vi "多参数测量数据读取.vi"(8 "Error in":errorcluster caption="Error in (no error)", 11 "探头选择":u16(ring)=9 items=["氨氮"=3, "水温"=9, "pH值"=10, "溶解氧"=11, "电导率"=12, "浊度"=13, "叶绿素a"=14, "藻密度"=15, "蓝绿藻"=16, "氧化还原电位"=17, "溶解氧%"=18, "盐度"=19]) -> (0 "error out":errorcluster, 2 "添加的数组":string[][](array[string]), 3 "测量数据块":T1)   [LabVIEW 2016, in "斯坦道原位多参数.lvlib"]
panel:
  in  "测量数据区":i32(listbox)
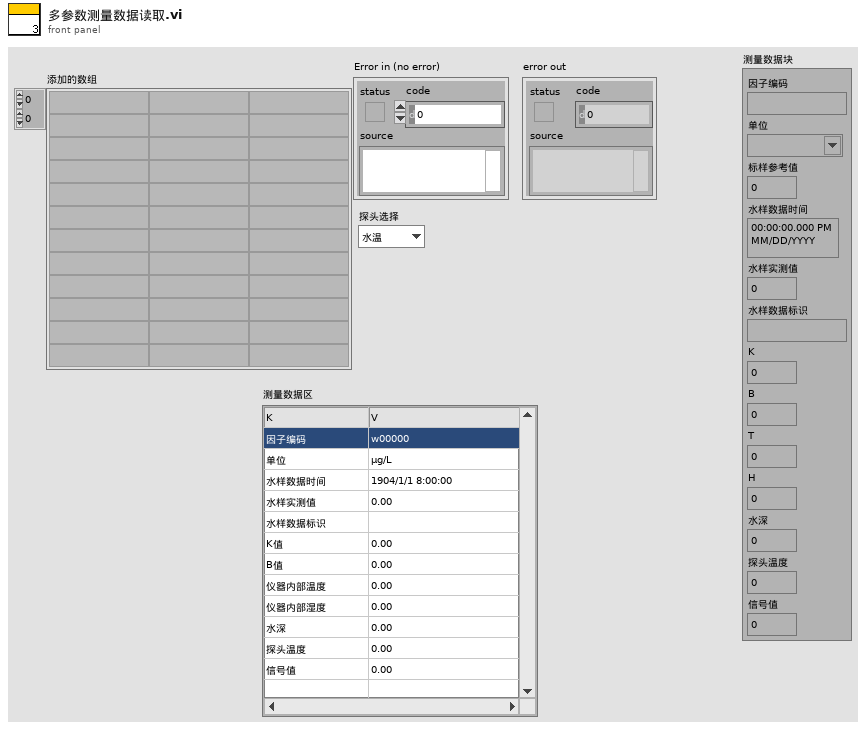
[diagram p1: front panel]
types:
  T1 = cluster{"因子编码":string, "单位":string, "标样参考值":sgl, "水样数据时间":timestamp, "水样实测值":sgl, "水样数据标识":string, "K":sgl, "B":sgl, "T":sgl, "H":sgl, "水深":sgl, "探头温度":sgl, "信号值":sgl}
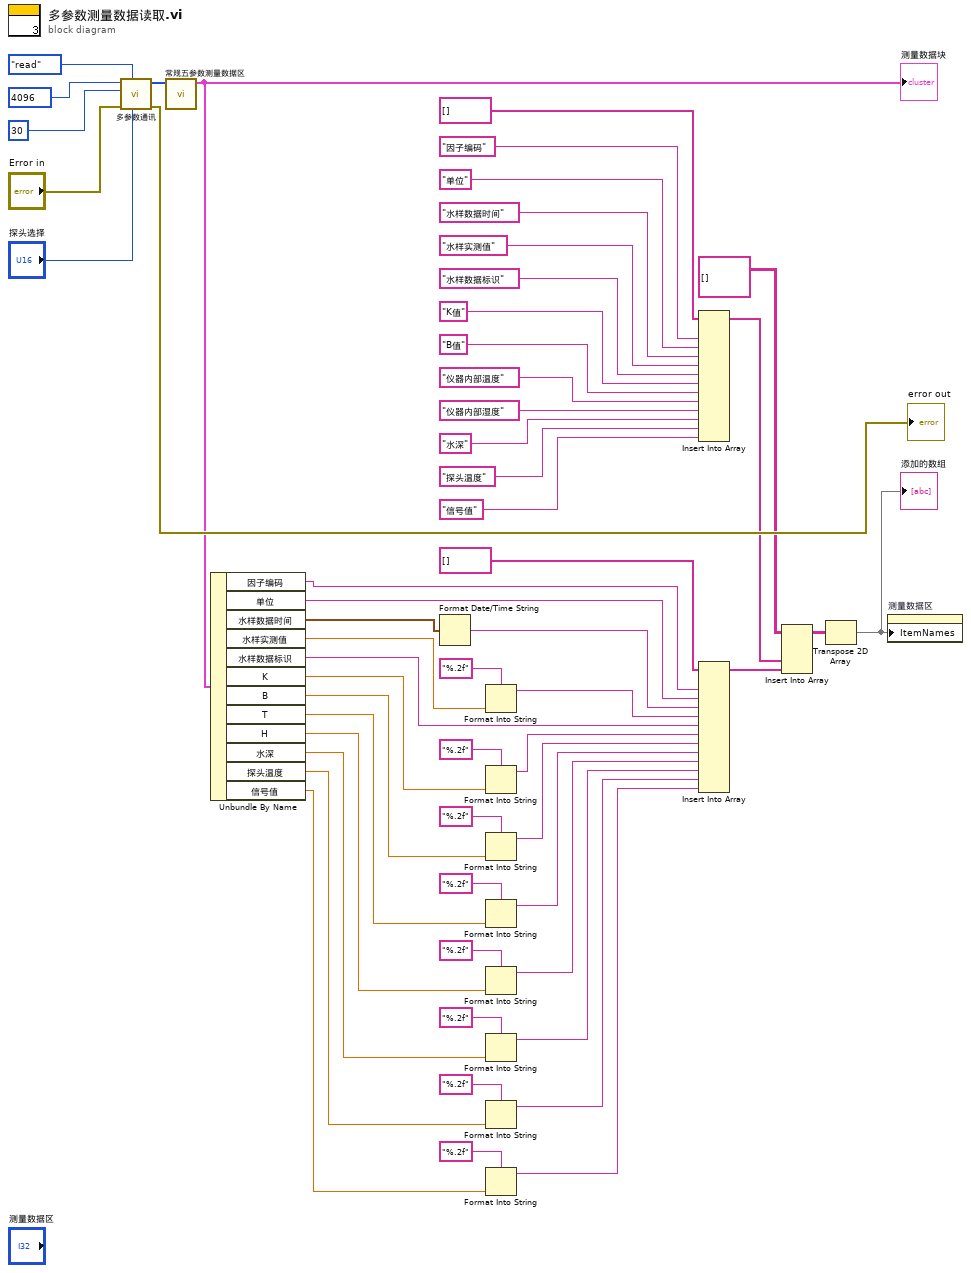
[diagram p0: block diagram]
diagram:
  n1 = call "多参数通讯.vi"("Slave ID"="探头选择", "STEP"=enum16{"open", "read", "write", "close"}."read", "Error in"="Error in", "quantity"=u16 30, "starting address"=u16 4096) -> ("error out"=→"error out":errorcluster, "Registers"=w47:u16[])  [unwired: 4 in, 1 out]
  n2 = call "常规五参数测量数据区.vi"("数组"=w47) -> ("测量数据区"=w27:T1)  [unwired: 10 in]
  "测量数据块" <- w27
  n3 = Unbundle By Name(w27) -> ("因子编码"=w26:string, "单位"=w25:string, "水样数据时间"=w24:timestamp, "水样实测值"=w23:sgl, "水样数据标识"=w22:string, "K"=w20:sgl, "B"=w14:sgl, "T"=w13:sgl, "H"=w12:sgl, "水深"=w11:sgl, "探头温度"=w10:sgl, "信号值"=w3:sgl)
  n4 = Format Date/Time String(seconds (now)=w24) -> (date/time string=w49:string)  [unwired: 2 in]
  n5 = Format Into String(format string="%.2f" ("格式字符串"), w23) -> (resulting string=w48:string)  [unwired: 2 in, 1 out]
  n6 = Format Into String(format string="%.2f" ("格式字符串"), w20) -> (resulting string=w9:string)  [unwired: 2 in, 1 out]
  n7 = Format Into String(format string="%.2f" ("格式字符串"), w14) -> (resulting string=w8:string)  [unwired: 2 in, 1 out]
  n8 = Format Into String(format string="%.2f" ("格式字符串"), w13) -> (resulting string=w7:string)  [unwired: 2 in, 1 out]
  n9 = Format Into String(format string="%.2f" ("格式字符串"), w12) -> (resulting string=w6:string)  [unwired: 2 in, 1 out]
  n10 = Format Into String(format string="%.2f" ("格式字符串"), w11) -> (resulting string=w5:string)  [unwired: 2 in, 1 out]
  n11 = Format Into String(format string="%.2f" ("格式字符串"), w10) -> (resulting string=w2:string)  [unwired: 2 in, 1 out]
  n12 = Format Into String(format string="%.2f" ("格式字符串"), w3) -> (resulting string=w1:string)  [unwired: 2 in, 1 out]
  n13 = Insert Into Array(array=string[] [], new element #1="因子编码", new element #2="单位", new element #3="水样数据时间", new element #4="水样实测值", new element #5="水样数据标识", new element #6="K值", new element #7="B值", new element #8="仪器内部温度", new element #9="仪器内部湿度", new element #10="水深", new element #11="探头温度", new element #12="信号值") -> (w35:string[])  [unwired: 1 in]
  n14 = Insert Into Array(array=string[] [] ("数组"), new element #1=w26, new element #2=w25, new element #3=w49, new element #4=w48, new element #5=w22, new element #6=w9, new element #7=w8, new element #8=w7, new element #9=w6, new element #10=w5, new element #11=w2, new element #12=w1) -> (w34:string[])  [unwired: 1 in]
  n15 = Insert Into Array(array=string[][] [], new element #1=w35, new element #2=w34) -> (w33:string[][])  [unwired: 2 in]
  n16 = Transpose 2D Array(2D array=w33) -> (transposed array=w54:string[][])
  "添加的数组" <- w54
  n17 = property on="测量数据区" class="MCListbox (严格)"("ItemNames"=w54) -> ()  [unwired: 2 in, 2 out]
